vi "Write INI Tokens and VI Tags.vi"(8 "error in":errorcluster, 11 "Global Data in":T1={"Class"={"Ants"=refnum, "Layer"=refnum, "Templates"=refnum, "Icon"=refnum, "Glyph"=refnum, "Settings"=refnum, "Tools"=refnum}, "Ref"={"Add Layer"=refnum, "Remove Layer"=refnum, "Line Text"=[], "Body Text Spec"=refnum, "DNL_Font"=refnum, "glyph path str"=refnum, "templates path str"=refnum, "Arrow Up"=refnum, "Arrow Down"=refnum, "IE VI Ref"=refnum, "Glyphs tree"=refnum, "Templates tree"=refnum, "Layer Icon Text"=refnum, "Layer Template"=refnum, "Body Text"=refnum, "Search Templates"=refnum, "TextMarker"=refnum, "Tab Control"=refnum, "Search Glyphs"=refnum, "Line Color"=refnum, "DNL_Glyphs []"=refnum, "Fill Color"=refnum, "Tools"=refnum, "Icon"=refnum, "Preview"=refnum, "Ants"=refnum, "Terminals"=refnum, "menu reference"=refnum, "LayerNames"=[], "GlyphLoadAnimation"=refnum, "TemplateLoadAnimation"=refnum, "refreshGlyphs"=refnum, "refreshTemplates"=refnum}, "Support"={"AntsRect"={"left"=0, "top"=0, "right"=0, "bottom"=0}, "Mouse Move Coords"={"Horizontal"=0, "Vertical"=0}, "Mouse Down Coords"={"Horizontal"=0, "Vertical"=0}, "Temp Coord"={"Horizontal"=0, "Vertical"=0}, "Action"=enum."Default", "Edge Color"=4914962, "Fill Color"=16860, "Mouse Down?"=FALSE, "Draft Mode?"=FALSE, "Temp Icon"=bytes[3102], "CTRL Pressed"=FALSE, "Move Selection?"=FALSE, "AntsRect Orig"={"left"=0, "top"=0, "right"=0, "bottom"=0}, "Text"="", "TM Set?"=FALSE, "Mouse inside icon?"=FALSE, "Tool (old value)"=0, "Pencil Move Color"=0, "Swap Colors?"=FALSE, "Shift pressed?"=FALSE}}) -> (0 "error out":errorcluster, 3 "Global Data out":T1={"Class"={"Ants"=refnum, "Layer"=refnum, "Templates"=refnum, "Icon"=refnum, "Glyph"=refnum, "Settings"=refnum, "Tools"=refnum}, "Ref"={"Add Layer"=refnum, "Remove Layer"=refnum, "Line Text"=[], "Body Text Spec"=refnum, "DNL_Font"=refnum, "glyph path str"=refnum, "templates path str"=refnum, "Arrow Up"=refnum, "Arrow Down"=refnum, "IE VI Ref"=refnum, "Glyphs tree"=refnum, "Templates tree"=refnum, "Layer Icon Text"=refnum, "Layer Template"=refnum, "Body Text"=refnum, "Search Templates"=refnum, "TextMarker"=refnum, "Tab Control"=refnum, "Search Glyphs"=refnum, "Line Color"=refnum, "DNL_Glyphs []"=refnum, "Fill Color"=refnum, "Tools"=refnum, "Icon"=refnum, "Preview"=refnum, "Ants"=refnum, "Terminals"=refnum, "menu reference"=refnum, "LayerNames"=[], "GlyphLoadAnimation"=refnum, "TemplateLoadAnimation"=refnum, "refreshGlyphs"=refnum, "refreshTemplates"=refnum}, "Support"={"AntsRect"={"left"=0, "top"=0, "right"=0, "bottom"=0}, "Mouse Move Coords"={"Horizontal"=0, "Vertical"=0}, "Mouse Down Coords"={"Horizontal"=0, "Vertical"=0}, "Temp Coord"={"Horizontal"=0, "Vertical"=0}, "Action"=enum."Default", "Edge Color"=4914962, "Fill Color"=16860, "Mouse Down?"=FALSE, "Draft Mode?"=FALSE, "Temp Icon"=bytes[3102], "CTRL Pressed"=FALSE, "Move Selection?"=FALSE, "AntsRect Orig"={"left"=0, "top"=0, "right"=0, "bottom"=0}, "Text"="", "TM Set?"=FALSE, "Mouse inside icon?"=FALSE, "Tool (old value)"=0, "Pencil Move Color"=0, "Swap Colors?"=FALSE, "Shift pressed?"=FALSE}})   [LabVIEW 2021]
uses:
  <resource>/plugins/NIIconEditor/Class/Ants/Ants.lvclass
  <resource>/plugins/NIIconEditor/Class/FakedArray/FakedArray.lvclass
  <vilib>/LabVIEW Icon API/lv_icon/Classes/Icon/Icon.lvclass
  <resource>/plugins/NIIconEditor/Class/Icon Library/Glyph.lvclass
  <resource>/plugins/NIIconEditor/Class/Settings/Settings.lvclass
  <resource>/plugins/NIIconEditor/Class/Tools/Tools Paint.lvclass
  <vilib>/LabVIEW Icon API/lv_icon/Classes/Icon Framework/Icon Framework.lvclass
  <vilib>/LabVIEW Icon API/lv_icon/Classes/Layer/Layer.lvclass
  <vilib>/LabVIEW Icon API/lv_icon/lv_icon.lvlib
  <vilib>/LabVIEW Icon API/lv_icon/Controls/Font.ctl
  <vilib>/LabVIEW Icon API/lv_icon/Controls/Alignment.ctl
  <resource>/plugins/NIIconEditor/Controls/Font Size.ctl
  <vilib>/LabVIEW Icon API/lv_icon/Controls/BodyText.ctl
  <vilib>/LabVIEW Icon API/lv_icon/Controls/IEColor.ctl
  <resource>/plugins/NIIconEditor/Controls/Tools.ctl
  <resource>/plugins/NIIconEditor/INI/INI Data.ctl
  <vilib>/Utility/miscctls.llb/LVPoint32TypeDef.ctl
  <resource>/plugins/NIIconEditor/Controls/SupportClass_Action.ctl
  <resource>/plugins/NIIconEditor/Controls/SupportClass.ctl
  <resource>/plugins/NIIconEditor/Controls/References Cluster.ctl
  <resource>/plugins/NIIconEditor/Controls/IE Classes.ctl
  <resource>/plugins/NIIconEditor/Controls/Global Data.ctl
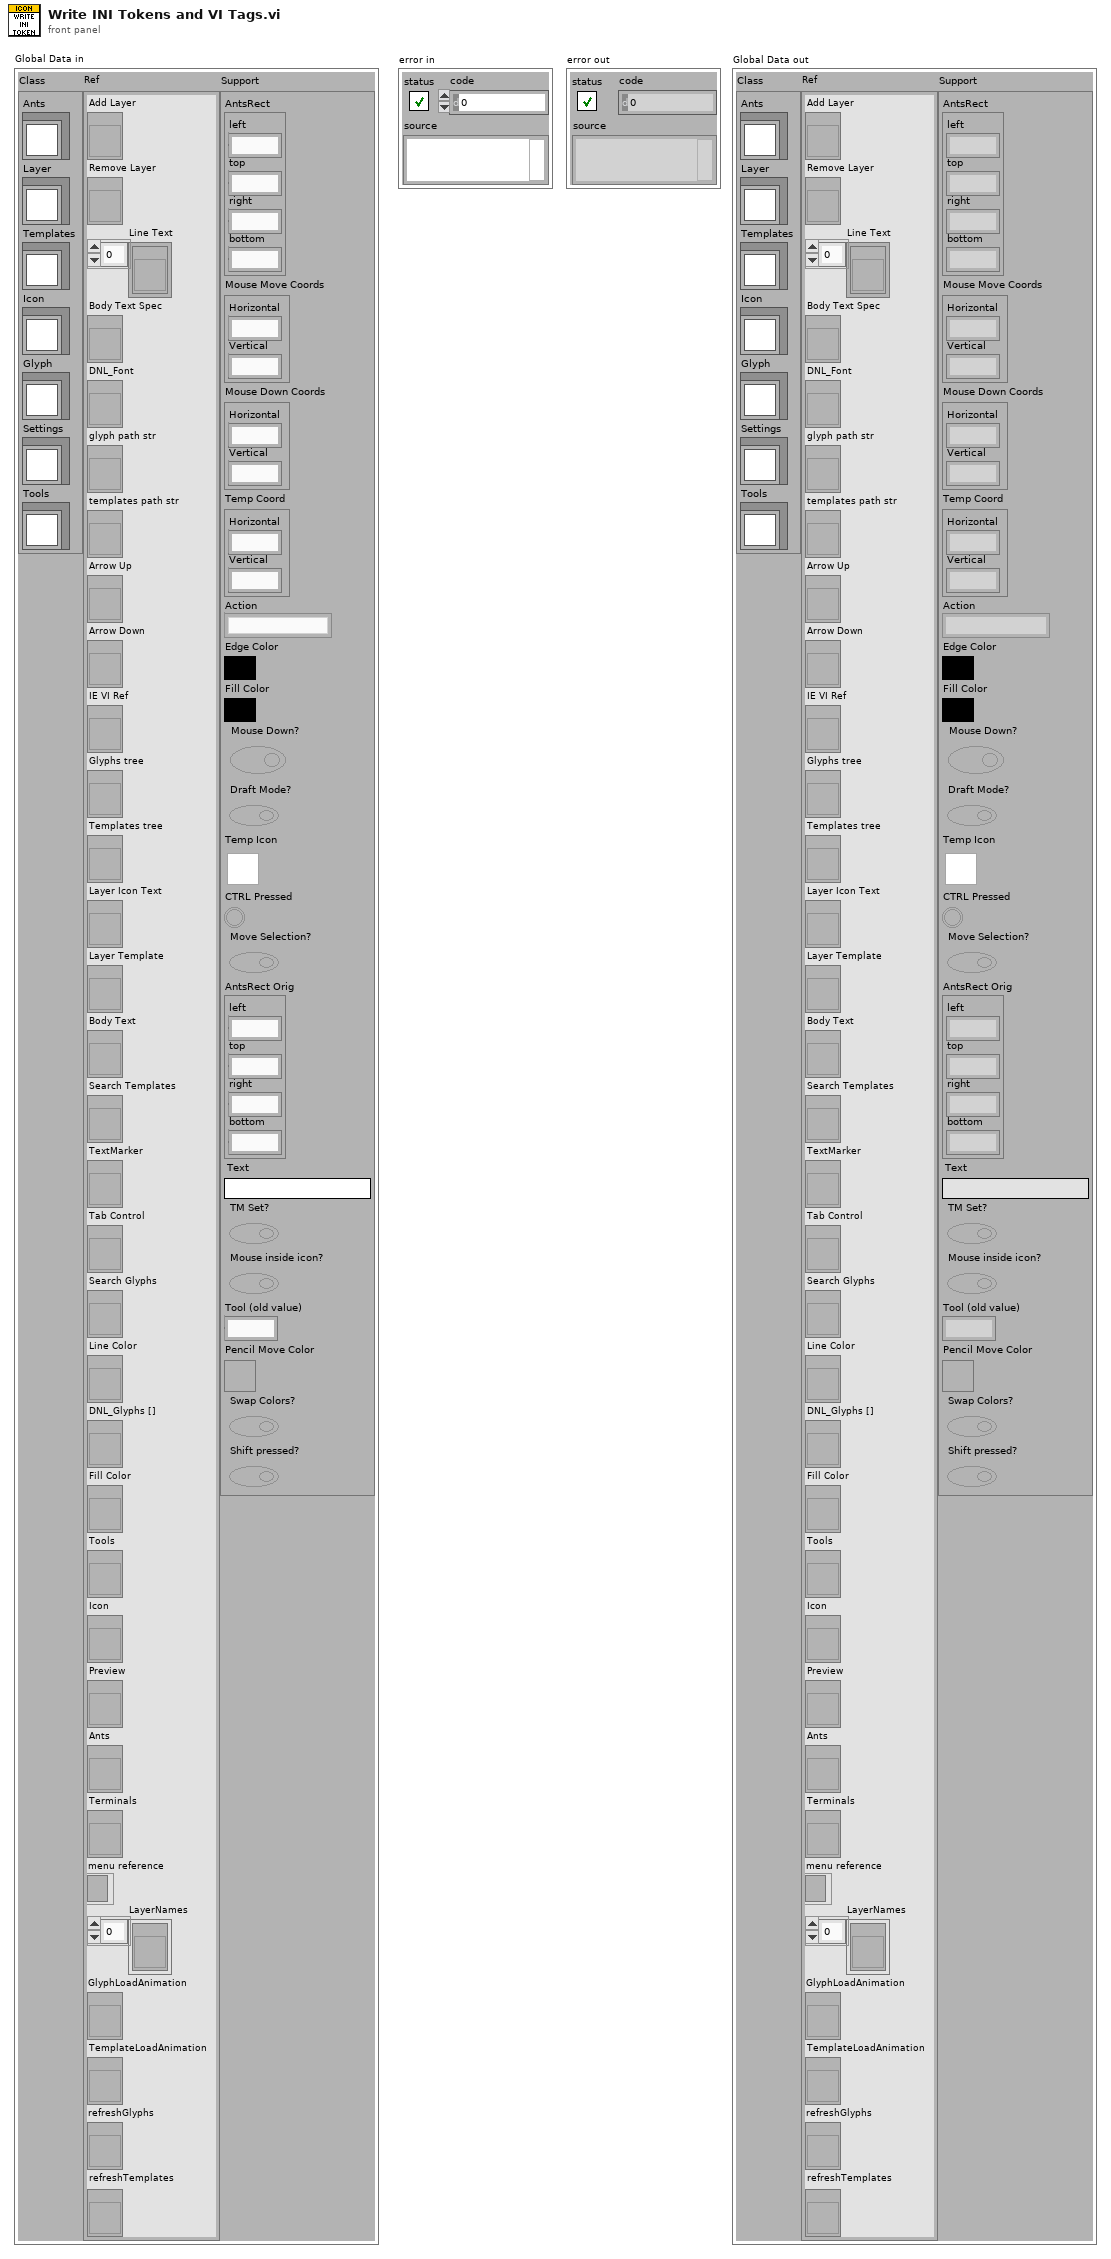
[diagram p1: front panel]
types:
  T1 = typedef "lv_icon.lvlib/Global Data.ctl" = cluster{"Class":T2, "Ref":T3, "Support":T4}
  T2 = typedef "IE Classes.ctl" = cluster{"Ants":refnum<class "Ants.lvclass">, "Layer":refnum<class "FakedArray.lvclass">, "Templates":refnum<class "FakedArray.lvclass">, "Icon":refnum<class "Icon.lvclass">, "Glyph":refnum<class "Glyph.lvclass">, "Settings":refnum<class "Settings.lvclass">, "Tools":refnum<class "Tools Paint.lvclass">}
  T3 = typedef "lv_icon.lvlib/References Cluster.ctl" = cluster{"Add Layer":refnum<vi>, "Remove Layer":refnum<vi>, "Line Text":refnum<vi>[], "Body Text Spec":refnum<vi>, "DNL_Font":refnum<vi>, "glyph path str":refnum<vi>, "templates path str":refnum<vi>, "Arrow Up":refnum<vi>, "Arrow Down":refnum<vi>, "IE VI Ref":refnum<vi>, "Glyphs tree":refnum<vi>, "Templates tree":refnum<vi>, "Layer Icon Text":refnum<vi>, "Layer Template":refnum<vi>, "Body Text":refnum<vi>, "Search Templates":refnum<vi>, "TextMarker":refnum<vi>, "Tab Control":refnum<vi>, "Search Glyphs":refnum<vi>, "Line Color":refnum<vi>, "DNL_Glyphs []":refnum<vi>, "Fill Color":refnum<vi>, "Tools":refnum<vi>, "Icon":refnum<vi>, "Preview":refnum<vi>, "Ants":refnum<vi>, "Terminals":refnum<vi>, "menu reference":refnum<k9>, "LayerNames":refnum<vi>[], "GlyphLoadAnimation":refnum<vi>, "TemplateLoadAnimation":refnum<vi>, "refreshGlyphs":refnum<vi>, "refreshTemplates":refnum<vi>}
  T4 = typedef "SupportClass.ctl" = cluster{"AntsRect":cluster{"left":i16, "top":i16, "right":i16, "bottom":i16}, "Mouse Move Coords":T5, "Mouse Down Coords":T5, "Temp Coord":T5, "Action":T6, "Edge Color":T7, "Fill Color":T7, "Mouse Down?":bool, "Draft Mode?":bool, "Temp Icon":picture, "CTRL Pressed":bool, "Move Selection?":bool, "AntsRect Orig":cluster{"left":i16, "top":i16, "right":i16, "bottom":i16}, "Text":string, "TM Set?":bool, "Mouse inside icon?":bool, "Tool (old value)":u32, "Pencil Move Color":u32, "Swap Colors?":bool, "Shift pressed?":bool}
  T5 = typedef "LVPoint32TypeDef.ctl" = cluster{"Horizontal":i32, "Vertical":i32}
  T6 = typedef "SupportClass_Action.ctl" = enum16{"Default", "Move Selection", "Glyph Library", "Tool"}
  T7 = typedef "IEColor.ctl" = u32
  T8 = typedef "lv_icon.lvlib/INI Data.ctl" = cluster{"Show Terminals?":bool, "Text":cluster{"Font":T9, "Alignment":T10, "Size":T11}, "3rd party Templates":cluster{"Store 3rd party Templates?":bool, "Folder Name":string}, "Merge user layers on commit":bool, "Body Text":T12, "Fill Color":T7, "Edge Color":T7, "Tab":u16, "Tool":T13, "Disable Layers?":bool}
  T9 = typedef "Font.ctl" = string
  T10 = typedef "Alignment.ctl" = u16
  T11 = typedef "Font Size.ctl" = u8
  T12 = typedef "BodyText.ctl" = cluster{"Line 1 text":string, "Line 2 text":string, "Line 3 text":string, "Line 4 text":string, "Line 1 color":u32, "Line 2 color":u32, "Line 3 color":u32, "Line 4 color":u32, "Body Text Spec":cluster{"Font":T9, "Alignment":T10, "Size":u8}, "Center text vertically":bool, "Capitalize Text":bool}
  T13 = typedef "Tools.ctl" = enum32{"Pencil", "Line", "Dropper", "Fill", "Rectangle", "Filled Rectangle", "Ellipse", "Filled Ellipse", "Eraser", "Text", "Select", "Move"}
  T14 = enum32{"Pencil", "Line", "Dropper", "Fill", "Rectangle", "Filled Rectangle", "Ellipse", "Filled Ellipse", "Eraser", "Text", "Select", "Move"}
  T15 = typedef "LVRectTypeDef.ctl" = cluster{"Left":i16, "Top":i16, "Right":i16, "Bottom":i16}
  T16 = cluster{"LayerIcon":picture, "LayerName":string, "Opacity":u8, "Visibility?":bool}
  T17 = enum32{"Templates", "Icon Text", "Glyphs", "Layers"}
  T18 = typedef "Icon Editor Invoker Type.ctl" = enum32{"Unknown Icon Source", "VI Icon", "Library Icon (any library type)", "Palette icon", "Icon from App Method"}
  T19 = typedef "Pathes.ctl" = enum16{"Root Path", "Icon Templates", "Icon Templates VI", "Icon Templates Lib", "Glyphs"}
  T20 = typedef "Graphic.ctl" = cluster{"Rectangle":cluster{"left":i16, "top":i16, "right":i16, "bottom":i16}, "Path":path, "Image":picture, "Filter":string, "FileName":string}
  T21 = cluster{"Visibility?":bool, "Opacity":u8, "Visibility?":bool, "Opacity":u8, "Relative Path from 1 to 2":path, "Image":picture, "Layers out":refnum<class "Layer.lvclass">[], "Body Text":T12}
  T22 = cluster{"Same Folder Structure?":bool, "Folder Name":string}
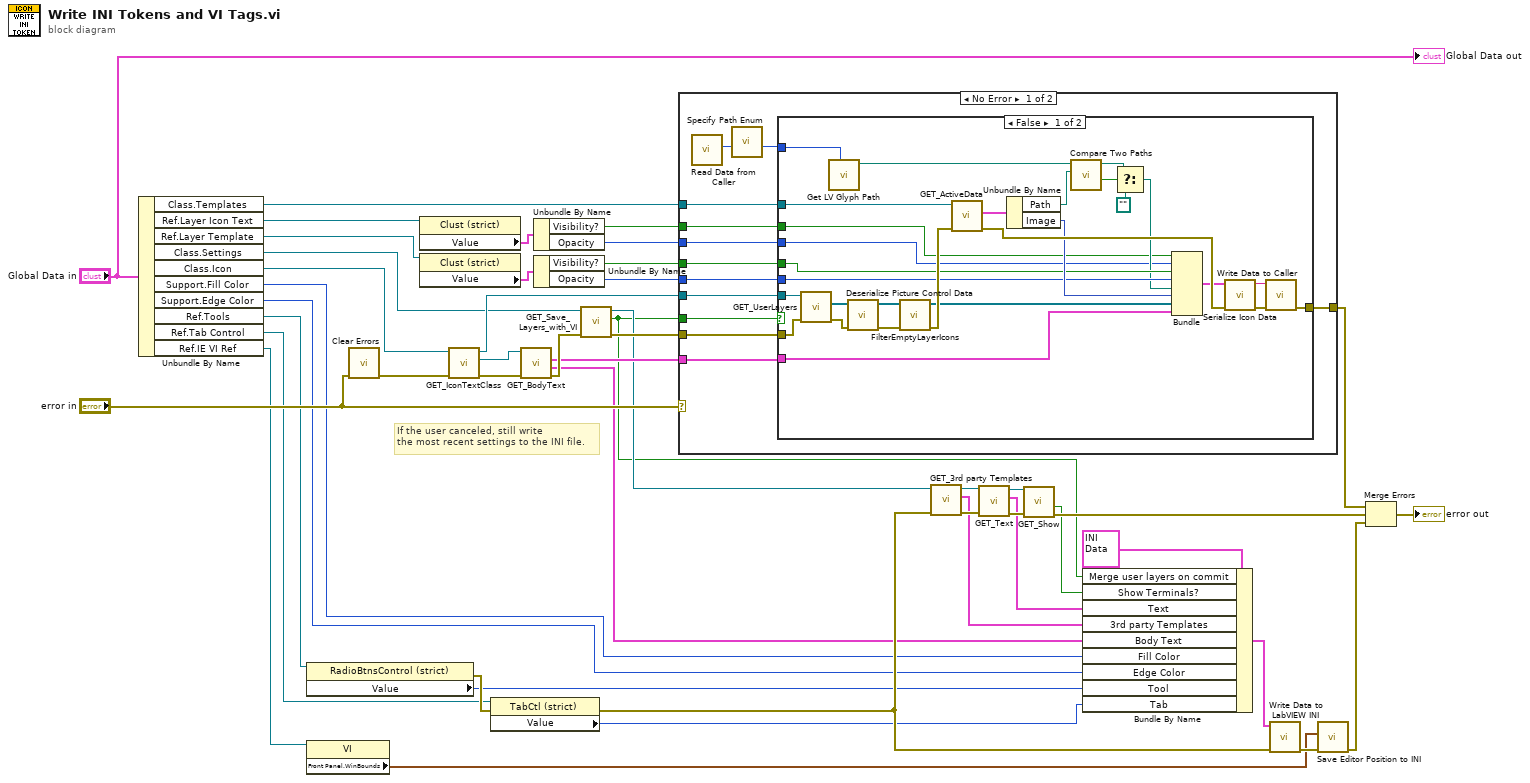
[diagram p0: block diagram]
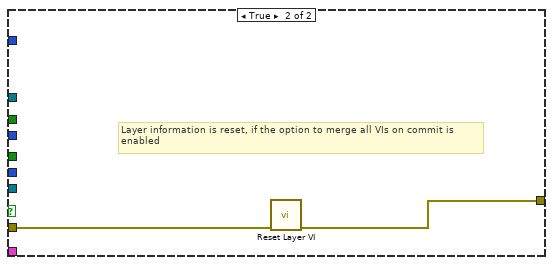
[diagram p2: hidden frame]
diagram:
  # "If the user canceled, still write\nthe most recent settings to the INI file."
  n1 = Unbundle By Name("Global Data in") -> ("Class.Templates"=w8:refnum<class "FakedArray.lvclass">, "Ref.Layer Icon Text"=w6:refnum<vi>, "Ref.Layer Template"=w14:refnum<vi>, "Class.Settings"=w16:refnum<class "Settings.lvclass">, "Class.Icon"=w15:refnum<class "Icon.lvclass">, "Support.Fill Color"=w13:T7, "Support.Edge Color"=w12:T7, "Ref.Tools"=w11:refnum<vi>, "Ref.Tab Control"=w10:refnum<vi>, "Ref.IE VI Ref"=w2:refnum<vi>)
  n2 = property class="RadioBtnsControl (strict)"(reference=w11) -> (error out=w41:errorcluster, "Value"=w24:T14)  [unwired: 1 in, 1 out]
  n3 = property class="VI"(reference=w2) -> ("Front Panel.WinBounds"=w1:T15)  [unwired: 1 in, 2 out]
  n4 = call <vilib>:"Clear Errors.vi"("error in (no error)"="error in") -> ("error out"=w40:errorcluster)  [unwired: 5 in, 1 out]
  n5 = property class="Clust (strict)"(reference=w6) -> ("Value"=w7:T16)  [unwired: 1 in, 2 out]
  n6 = property class="Clust (strict)"(reference=w14) -> ("Value"=w19:T16)  [unwired: 1 in, 2 out]
  n7 = call-dynamic "GET_IconTextClass.vi"("error in (no error)"=w40, "Icon.lvclass in"=w15) -> ("error out"=w45:errorcluster, "Icon Framework.lvclass"=w32:refnum<class "Icon Framework.lvclass">, "Icon.lvclass out"=w31:refnum<class "Icon.lvclass">)  [unwired: 7 out]
  n8 = property class="TabCtl (strict)"(reference=w10, error in=w41) -> (error out=w47:errorcluster, "Value"=w3:T17)  [unwired: 1 out]
  n9 = call-dynamic "GET_BodyText.vi"("error in (no error)"=w45, "Icon Framework.lvclass in"=w32) -> ("error out"=w46:errorcluster, "Cleaned Body Text"=w23:T12, "Body Text"=w30:T12)  [unwired: 7 out]
  n10 = Unbundle By Name(w7) -> ("Visibility?"=w4:bool, "Opacity"=w5:u8)
  n11 = Unbundle By Name(w19) -> ("Visibility?"=w17:bool, "Opacity"=w18:u8)
  n12 = call <resource>:"GET_Save_Layers_with_VI.vi"("error in (no error)"=w46, "Settings.lvclass in"=w16) -> ("error out"=w44:errorcluster, "Merge user layers on commit"=w9:bool, "Settings.lvclass out"=w29:refnum<class "Settings.lvclass">)  [unwired: 7 out]
  n13 = case shown="No Error" "error in" {
    selector: "error in" -> [_ w90]
    tunnel: [w59 w90] -> w37
    tunnel: w31 -> [w57 _]
    tunnel: w30 -> [w56 _]
    tunnel: w44 -> [w58 _]
    tunnel: w18 -> [w55 _]
    tunnel: w17 -> [w54 _]
    tunnel: w9 -> [w51 _]
    tunnel: w8 -> [w50 _]
    tunnel: w5 -> [w49 _]
    tunnel: w4 -> [w48 _]
    frame No Error {
      n14 = call <resource>:"Read Data from Caller.vi"() -> ("Icon Editor Invoker Type"=w53:T18)  [unwired: 3 in, 8 out]
      n15 = call <resource>:"Specify Path Enum.vi"("Icon Editor Invoker Type"=w53) -> ("Path"=w52:T19)  [unwired: 10 out]
      n16 = case shown="False" w51 {
        tunnel: w57 -> [w79 _]
        tunnel: w58 -> [w87 w89]
        tunnel: w56 -> [w77 _]
        tunnel: [w85 w88] -> w59
        tunnel: w52 -> [w73 _]
        tunnel: w50 -> [w72 _]
        tunnel: w55 -> [w71 _]
        tunnel: w54 -> [w70 _]
        tunnel: w49 -> [w62 _]
        tunnel: w48 -> [w61 _]
        frame False {
          n17 = call-dynamic "GET_UserLayers.vi"("error in (no error)"=w87, "Icon.lvclass in"=w79) -> ("error out"=w83:errorcluster, "All Layers"=w69:refnum<class "Layer.lvclass">[])  [unwired: 8 out]
          n18 = call <vilib>:"Get LV Glyph Path.vi"("Path"=w73) -> ("Requested Path"=w76:path)  [unwired: 2 in, 8 out]
          n19 = call <vilib>:"Deserialize Picture Control Data.vi"("error in (no error)"=w83, "Layers in"=w69) -> ("error out"=w82:errorcluster, "Layers out"=w64:refnum<class "Layer.lvclass">[])  [unwired: 8 out]
          n20 = call <vilib>:"FilterEmptyLayerIcons.vi"("error in (no error)"=w82, "Layers"=w64) -> ("error out"=w81:errorcluster, "Layers out"=w63:refnum<class "Layer.lvclass">[])  [unwired: 8 out]
          n21 = call-dynamic "GET_ActiveData.vi"("error in (no error)"=w81, "FakedArray in"=w72) -> ("error out"=w84:errorcluster, "Path & Icon"=w80:T20)  [unwired: 8 out]
          n22 = Unbundle By Name(w80) -> ("Path"=w75:path, "Image"=w78:picture)
          n23 = call <vilib>:"Compare Two Paths.vi"("Path 2"=w75, "Path 1"=w76) -> ("Path 2 Relative to Path 1?"=w68:bool, "Relative Path from 1 to 2"=w67:path)  [unwired: 1 in, 7 out]
          n24 = Select(t=w67, s=w68, f=path "") -> (s? t:f=w66:path)
          n25 = Bundle("Visibility?"=w61, "Opacity"=w62, "Visibility?"=w70, "Opacity"=w71, "Relative Path from 1 to 2"=w66, "Image"=w78, "Layers out"=w63, "Body Text"=w77) -> (w60:T21)  [unwired: 1 out]
          n26 = call <vilib>:"Serialize Icon Data.vi"("error in"=w84, "Icon data"=w60) -> ("error out"=w86:errorcluster, "data string"=w74:string)  [unwired: 8 out]
          n27 = call <resource>:"Write Data to Caller.vi"("error in (no error)"=w86, "Data"=w74) -> ("error out"=w85:errorcluster)  [unwired: 9 out]
        }
        frame True {
          # "Layer information is reset, if the option to merge all VIs on commit is\nenabled"
          n28 = call <resource>:"Reset Layer VI.vi"("error in (no error)"=w89) -> ("error out"=w88:errorcluster)  [unwired: 10 out]
        }
      }
    }
    frame Error {
    }
  }
  n29 = call-dynamic "GET_3rd party Templates.vi"("error in (no error)"=w47, "Settings.lvclass in"=w29) -> ("error out"=w43:errorcluster, "3rd party Templates"=w22:T22, "Settings.lvclass out"=w28:refnum<class "Settings.lvclass">)  [unwired: 7 out]
  n30 = call-dynamic "GET_Text.vi"("error in (no error)"=w43, "Settings.lvclass in"=w28) -> ("error out"=w42:errorcluster, "Text"=w21:cluster{"Font":T9, "Alignment":T10, "Size":T11}, "Settings.lvclass out"=w27:refnum<class "Settings.lvclass">)  [unwired: 7 out]
  n31 = call-dynamic "GET_Show.vi"("error in"=w42, "Settings.lvclass in"=w27) -> ("error out"=w36:errorcluster, "Show Terminals?"=w20:bool)  [unwired: 8 out]
  n32 = Bundle By Name(cluster=T8 {"Show Terminals?"=FALSE, "Text"={"Font"="", "Alignment"=0, "Size"=0}, "3rd party Templates"={"Store 3rd party Templates?"=FALSE, "Folder Name"=""}, "Merge user layers on commit"=FALSE, "Body Text"={"Line 1 text"="", "Line 2 text"="", "Line 3 text"="", "Line 4 text"="", "Line 1 color"=0, "Line 2 color"=0, "Line 3 color"=0, "Line 4 color"=0, "Body Text Spec"={"Font"="", "Alignment"=0, "Size"=3}, "Center text vertically"=FALSE, "Capitalize Text"=FALSE}, "Fill Color"=0, "Edge Color"=0, "Tab"=0, "Tool"=enum."Ellipse", "Disable Layers?"=FALSE}, "Merge user layers on commit"=w9, "Show Terminals?"=w20, "Text"=w21, "3rd party Templates"=w22, "Body Text"=w23, "Fill Color"=w13, "Edge Color"=w12, "Tool"=w24, "Tab"=w3) -> (w26:T8)
  n33 = call <resource>:"Write Data to LabVIEW INI.vi"("error in"=w47, "INI Data"=w26) -> ("error out"=w38:errorcluster)  [unwired: 9 out]
  n34 = call <resource>:"Save Editor Position to INI.vi"("error in"=w38, "Window Bounds"=w1) -> ("error out"=w35:errorcluster)  [unwired: 9 in]
  n35 = Merge Errors(w37, w36, w35) -> (→"error out":errorcluster)
  "Global Data out" <- "Global Data in"
